vi "Actor Core.vi"(8 "error in":errorcluster, 11 "Chat Window Controller in":refnum<class "Chat Window UI Controller.lvclass">) -> (0 "error out":errorcluster, 3 "Actor out":refnum<class "Actor.lvclass">)   [LabVIEW 2020, in "Chat Window UI Controller.lvlib" / "Chat Window UI Controller.lvclass"]
doc: "(<B>Filename</B>: Actor Framework.lvlib:Actor.lvclass:Actor Core.vi)\n\nReceives messages to the actor, reacts to them, and initiates any error handling that may shut the actor down.\n\nDescendant classes may override this VI to append parallel tasks for the actor to complete while it handles messages. Overrides use the Call Parent Class Method node."
uses:
  Chat Window UI Controller.lvclass
  <vilib>/ActorFramework/Actor/Actor.lvclass
  Chat Window UI Controller.lvclass/Chat Window UI Controller.ctl
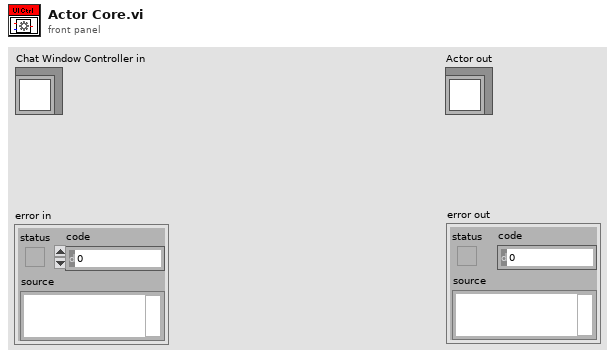
[diagram p1: front panel]
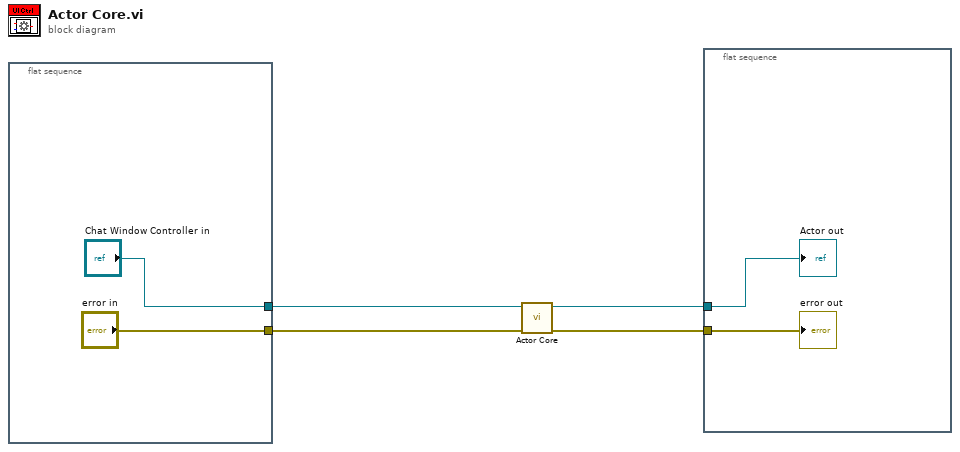
[diagram p0: block diagram]
diagram:
  n1 = flat-sequence {
    tunnel: ["error in"] -> w2
    tunnel: ["Chat Window Controller in"] -> w1
    frame #0 {
    }
  }
  n2 = call-parent "Actor Core.vi"("error in"=w2, "Actor in"=w1) -> ("error out"=w4:errorcluster, "Actor out"=w3:refnum<class "Actor.lvclass">)  [unwired: 8 in]
  n3 = flat-sequence {
    tunnel: w4 -> [w8]
    tunnel: w3 -> [w7]
    frame #0 {
      "error out" <- w8
      "Actor out" <- w7
    }
  }
